vi "GlobalNumPlotChannels.vi"() -> ()   [LabVIEW 2013]
panel:
  in  "NumPlotChannels":i32=48
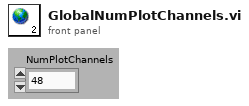
[diagram p1: front panel]
diagram:
